vi "Get Logging Event.vi"(8 "error in":errorcluster, 11 "UserEventHandler in":refnum<class "UserEventHandler.lvclass">) -> (0 "error out":errorcluster, 2 "Logging Event":refnum<user-event>, 3 "UserEventHandler out":refnum<class "UserEventHandler.lvclass">)   [LabVIEW 2016, in "hse-logger.lvlib" / "UserEventHandler.lvclass"]
doc: "Returns the ``Logging Event`` from the object. This ``Logging Event`` can be registered in any Event Structure.\n\n____\n(c) HAMPEL SOFTWARE ENGINEERING"
uses:
  UserEventHandler.lvclass
  LogRecord/LogRecord.lvclass
  UserEventHandler.lvclass/UserEventHandler.ctl
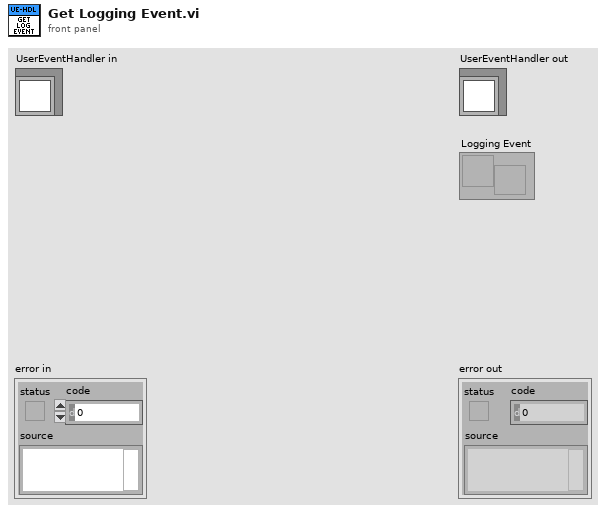
[diagram p1: front panel]
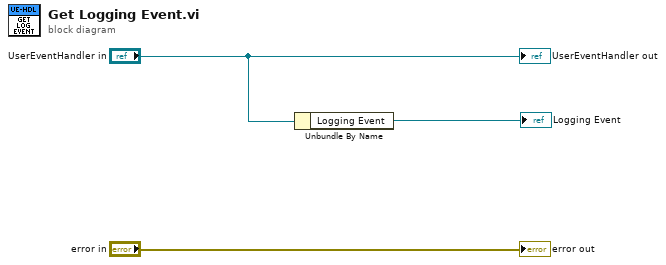
[diagram p0: block diagram]
diagram:
  n1 = Unbundle By Name("UserEventHandler in") -> ("Logging Event"=→"Logging Event":refnum<user-event>)
  "error out" <- "error in"
  "UserEventHandler out" <- "UserEventHandler in"
